vi "WSVCAP SHL Host TL RFFE Configure.vi"(7 "RFFE Slave Address":u8=144 caption="Slave Address" format="0x%02x", 9 "Clock Rate (Hz)":dbl=50000.0, 11 "error in":errorcluster, 13 "Log (T)":bool=TRUE) -> (6 "Actual Rate (Hz)":dbl, 15 "error out":errorcluster)   [LabVIEW 2012]
uses:
  Type Defs/WSVCAP SHL Function Enum.ctl
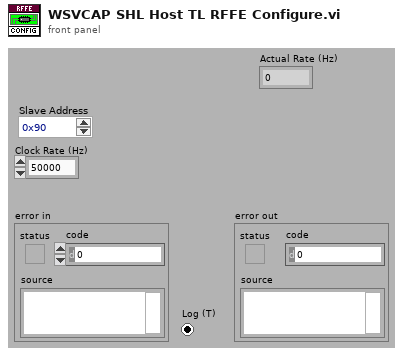
[diagram p1: front panel]
types:
  T1 = typedef "WSVCAP SHL Function Enum.ctl" = enum16{"Initialize", "Configure I2C", "Configure SPI", "Configure RFFE", "Write I2C", "Read I2C", "Write/Read SPI", "Start SPI Cycle", "Stop SPI Cycle", "Write RFFE", "Read RFFE", "Start RFFE Cycle", "Stop RFFE Cycle", "Get Status", "Close"}
  T2 = typedef "WSVCAP SHL Core System Cluster.ctl" = cluster{"Settings":T3, "FPGA Resource":tag, "Online":bool, "I2C Wait Ticks":u32, "SPI Wait Ticks":u32, "RFFE Wait Ticks":u32}
  T3 = typedef "WSVCAP SHL I2C Settings Cluster.ctl" = cluster{"FPGA Resource Name":string, "I2C Slave Address":u8, "I2C Clock Rate (Hz)":dbl, "SPI Clock Rate (Hz)":dbl, "RFFE Slave Address":u8, "RFFE Clock Rate (Hz)":dbl, "Simulate FPGA":bool}
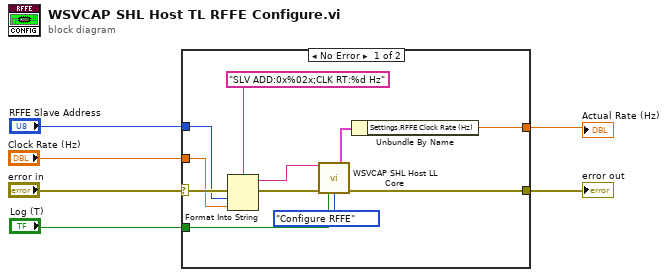
[diagram p0: block diagram]
diagram:
  n1 = case shown="No Error" "error in" {
    selector: "error in" -> [w13 w18]
    tunnel: [w17 w18] -> w6
    tunnel: [w15 _] -> w5
    tunnel: "Clock Rate (Hz)" -> [w11 _]
    tunnel: "Log (T)" -> [w9 _]
    tunnel: "RFFE Slave Address" -> [w7 _]
    frame No Error {
      n2 = Format Into String(format string="SLV ADD:0x%02x;CLK RT:%d Hz", error in=w13, w7, w11) -> (resulting string=w10:string, error out=w12:errorcluster)  [unwired: 1 in]
      n3 = call "WSVCAP SHL Host LL Core.vi"("Message In"=w10, "error in"=w12, "Log (T)"=w9, "Function"=WSVCAP_SHL_Function_Enum."Configure RFFE") -> ("System"=w16:T2, "error out"=w17:errorcluster)  [unwired: 9 in, 1 out]
      n4 = Unbundle By Name(w16) -> ("Settings.RFFE Clock Rate (Hz)"=w15:dbl)
    }
    frame Error {
    }
  }
  "Actual Rate (Hz)" <- w5
  "error out" <- w6
